vi "Close.vi"(8 "error in (no error)":errorcluster, 11 "Pump Calibration Config in":T1={"Settings"={"Cycle Period"=500.0, "Ismatech"={"VISA resource name"="", "Simulated?"=TRUE, "Pump Number"=1.0, "Reverse?"=FALSE}, "Masterflex"={"VISA resource name"="", "Simulated?"=TRUE, "Pump Number"=1.0, "Reverse?"=FALSE}, "Bronkhorst M13 Flow Meter"={"VISA resource name"="", "Simulated?"=TRUE}, "PID 2 Parameters"={"Input Device"=enum."Default", "Output Device"=enum."Default"}, "Bronkhorst M14"={"VISA resource name"="", "Simulated?"=FALSE}, "Tacmina Settings"={"Analog DAQ Task"="", "Digital DAQ Task"=""}, "KNF SIMDOS Settings"={"VISA resource name"="", "Simulated?"=TRUE}, "VICI M50 Settings"={"VISA resource name"="", "Simulated?"=TRUE, "Pump Letter"="", "Reverse?"=FALSE}, "FLOM Settings"={"VISA resource name"="", "Simulated?"=TRUE, "Pump Number"=0.0}, "Calibration Limits"={"Minimum (ml/min)"=0.0, "Maximum (ml/min)"=0.0, "Steps"=0.0}, "SSI PR Settings"={"VISA resource name"="", "Simulated?"=FALSE}}, "Flowmeter Output"=0.0, "Density"=0.0, "FL Temp"=0.0, "Speed %"=0.0, "File Refnum"=refnum, "Pump On?"=enum."Not Initialized"} {"Settings"."Masterflex"."Pump Number" min=1.0 max=20.0 step=1.0; "Settings"."Ismatech"."Pump Number" min=1.0 max=20.0 step=1.0}) -> (0 "error out":errorcluster, 3 "Pump Calibration Config out":T1={"Settings"={"Cycle Period"=500.0, "Ismatech"={"VISA resource name"="", "Simulated?"=TRUE, "Pump Number"=1.0, "Reverse?"=FALSE}, "Masterflex"={"VISA resource name"="", "Simulated?"=TRUE, "Pump Number"=1.0, "Reverse?"=FALSE}, "Bronkhorst M13 Flow Meter"={"VISA resource name"="", "Simulated?"=TRUE}, "PID 2 Parameters"={"Input Device"=enum."Default", "Output Device"=enum."Default"}, "Bronkhorst M14"={"VISA resource name"="", "Simulated?"=FALSE}, "Tacmina Settings"={"Analog DAQ Task"="", "Digital DAQ Task"=""}, "KNF SIMDOS Settings"={"VISA resource name"="", "Simulated?"=TRUE}, "VICI M50 Settings"={"VISA resource name"="", "Simulated?"=TRUE, "Pump Letter"="", "Reverse?"=FALSE}, "FLOM Settings"={"VISA resource name"="", "Simulated?"=TRUE, "Pump Number"=0.0}, "Calibration Limits"={"Minimum (ml/min)"=0.0, "Maximum (ml/min)"=0.0, "Steps"=0.0}, "SSI PR Settings"={"VISA resource name"="", "Simulated?"=FALSE}}, "Flowmeter Output"=0.0, "Density"=0.0, "FL Temp"=0.0, "Speed %"=0.0, "File Refnum"=refnum, "Pump On?"=enum."Not Initialized"} {"Settings"."Masterflex"."Pump Number" min=1.0 max=20.0 step=1.0; "Settings"."Ismatech"."Pump Number" min=1.0 max=20.0 step=1.0})   [LabVIEW 2018, in "Calibration.lvlib" / "Engine.lvlib"]
uses:
  Engine.lvlib
  Pump Calibration Config.ctl
  Pfizer Timed Seq/Software/Ismatec ISM 831C/Controls/Ismatech Settings Cluster.ctl
  Pfizer Timed Seq/Software/Masterflex 7550-30/Controls/Settings Cluster.ctl
  Pfizer Timed Seq/Software/Bronkhorst M13 Flow Meter/Settings Cluster.ctl
  Pfizer Timed Seq/Software/Measure Instrument/PID Input Enum.ctl
  Pfizer Timed Seq/Software/Measure Instrument/PID 2 Output Enum.ctl
  Pfizer Timed Seq/Software/Mettler Toledo/Controls/Settings Cluster.ctl
  Pfizer Timed Seq/Software/Tacmina QI/Tacmina QI DAQ Setting.ctl
  Pfizer Timed Seq/Software/KNF Pump/Settings Cluster plus SIMDOS.ctl
  Pfizer Timed Seq/Software/VICI M50 Party Mode/Settings Cluster.ctl
  Pfizer Timed Seq/Software/FLOM Pump/Settings Cluster.ctl
  Pfizer Timed Seq/Software/SSI PR Class/SSI PR Settings Cluster.ctl
  Pfizer Timed Seq/Software/Bronkhorst M13 Flow Meter/Bronkhorst M13 Flow Meter.lvlib
  Pfizer Timed Seq/Software/Bronkhorst M14 Flow Meter/Bronkhorst M14 Flow Meter.lvlib
  Pfizer Timed Seq/Software/Ismatec ISM 831C/Ismatec ISM 831C.lvlib
  Pfizer Timed Seq/Software/Masterflex 7550-30/Masterflex 7550-30.lvlib
  Pfizer Timed Seq/Software/VICI M50 Party Mode/VICI M6 M50 Party Mode.lvlib
  Pfizer Timed Seq/Software/Tacmina QI/Tacmina QI.lvlib
  Pfizer Timed Seq/Software/KNF Pump/KNF SIMDOS.lvlib
  Pfizer Timed Seq/Software/FLOM Pump/FLOM Pump.lvlib
  Pfizer Timed Seq/Software/SSI PR Class/SSI PR Pump.lvlib
  Pfizer Timed Seq/Software/Mettler Toledo/Mettler Toledo.lvlib
  Pfizer Timed Seq/Software/Calibration VIs/Calibration.lvlib
panel:
  # "Output Instruments"
  # "Input Instruments"
  # "Output Instruments"
  # "Input Instruments"
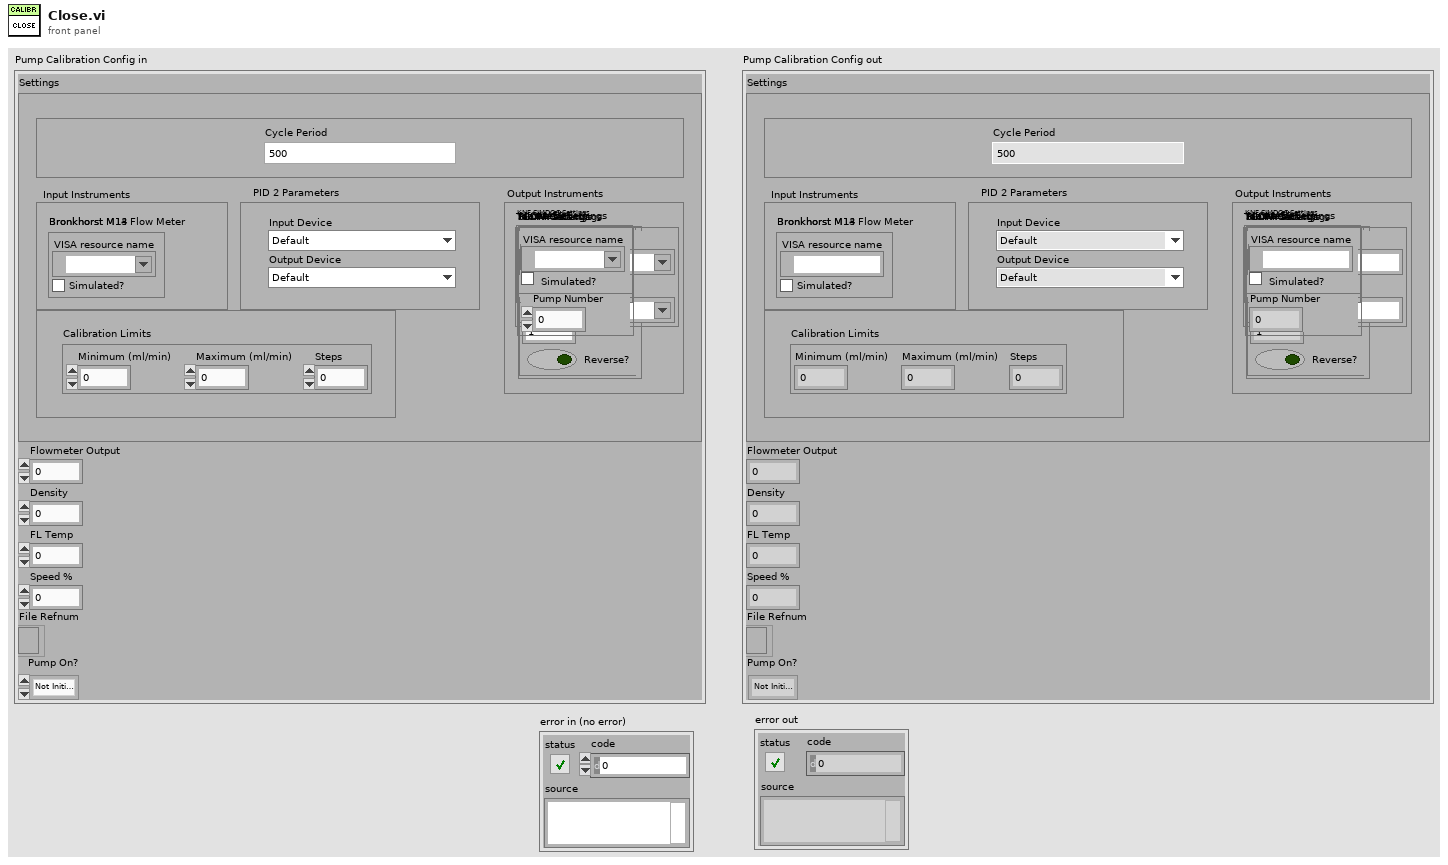
[diagram p1: front panel]
types:
  T1 = typedef "Calibration.lvlib/Pump Calibration Config.ctl" = cluster{"Settings":cluster{"Cycle Period":dbl, "Ismatech":T2, "Masterflex":T3, "Bronkhorst M13 Flow Meter":T4, "PID 2 Parameters":cluster{"Input Device":T5, "Output Device":T6}, "Bronkhorst M14":T7, "Tacmina Settings":T8, "KNF SIMDOS Settings":T9, "VICI M50 Settings":T10, "FLOM Settings":T11, "Calibration Limits":cluster{"Minimum (ml/min)":dbl, "Maximum (ml/min)":dbl, "Steps":dbl}, "SSI PR Settings":T12}, "Flowmeter Output":dbl, "Density":dbl, "FL Temp":dbl, "Speed %":dbl, "File Refnum":refnum<file>, "Pump On?":enum16{"Off", "On", "Not Initialized"}}
  T2 = typedef "Ismatec ISM 831C.lvlib/Ismatech Settings Cluster.ctl" = cluster{"VISA resource name":refnum<visa-resource-name>, "Simulated?":bool, "Pump Number":dbl, "Reverse?":bool}
  T3 = typedef "Masterflex 7550-30.lvlib/Settings Cluster.ctl" = cluster{"VISA resource name":refnum<visa-resource-name>, "Simulated?":bool, "Pump Number":dbl, "Reverse?":bool}
  T4 = typedef "Bronkhorst M13 Flow Meter.lvlib/Settings Cluster.ctl" = cluster{"VISA resource name":refnum<visa-resource-name>, "Simulated?":bool}
  T5 = typedef "PID Input Enum.ctl" = enum16{"Default", "Bronkhorst M13", "Bronkhorst M14", "Scale Rate of Change"}
  T6 = typedef "PID 2 Output Enum.ctl" = enum16{"Default", "Ismatec ISM 831C", "Masterflex 7550-30", "VICI", "Tacmina QI", "KNF SIMDOS", "ASIA Type C", "FLOM UI-22-11", "SSI PR"}
  T7 = typedef "Mettler Toledo.lvlib/Settings Cluster.ctl" = cluster{"VISA resource name":refnum<visa-resource-name>, "Simulated?":bool}
  T8 = typedef "Tacmina QI.lvlib/Tacmina QI DAQ Setting.ctl" = cluster{"Analog DAQ Task":refnum<k21>, "Digital DAQ Task":refnum<k21>}
  T9 = typedef "KNF SIMDOS.lvlib/Settings Cluster plus SIMDOS.ctl" = cluster{"VISA resource name":refnum<visa-resource-name>, "Simulated?":bool}
  T10 = typedef "VICI M6 M50 Party Mode.lvlib/Settings Cluster.ctl" = cluster{"VISA resource name":refnum<visa-resource-name>, "Simulated?":bool, "Pump Letter":string, "Reverse?":bool}
  T11 = typedef "FLOM Pump.lvlib/Settings Cluster.ctl" = cluster{"VISA resource name":refnum<visa-resource-name>, "Simulated?":bool, "Pump Number":dbl}
  T12 = typedef "SSI PR Pump.lvlib/SSI PR Settings Cluster.ctl" = cluster{"VISA resource name":refnum<visa-resource-name>, "Simulated?":bool}
  T13 = typedef "Bronkhorst M14 Flow Meter.lvlib/Settings Cluster.ctl" = cluster{"VISA resource name":refnum<visa-resource-name>, "Simulated?":bool}
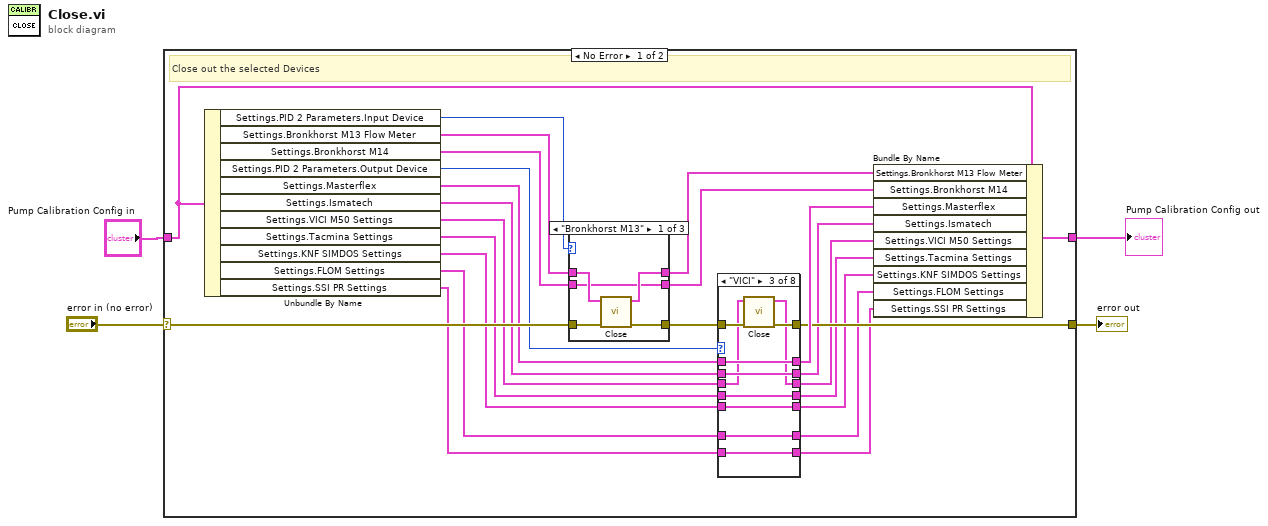
[diagram p0: block diagram]
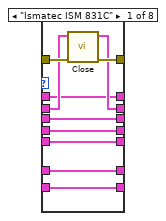
[diagram p2: hidden frame]
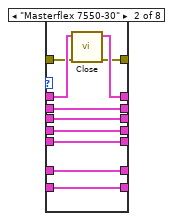
[diagram p3: hidden frame]
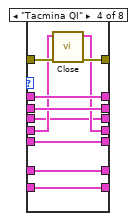
[diagram p4: hidden frame]
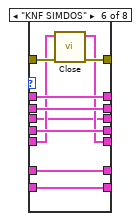
[diagram p6: hidden frame]
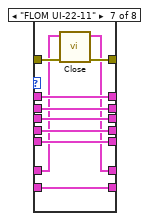
[diagram p7: hidden frame]
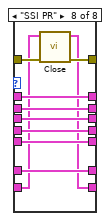
[diagram p8: hidden frame]
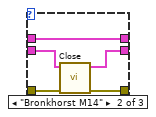
[diagram p9: hidden frame]
diagram:
  n1 = case shown="No Error" "error in (no error)" {
    selector: "error in (no error)" -> [w27 w122]
    tunnel: [w21 w122] -> w3
    tunnel: "Pump Calibration Config in" -> [w11 w121]
    tunnel: [w25 w121] -> w2
    frame No Error {
      # "Close out the selected Devices"
      n2 = Unbundle By Name(w11) -> ("Settings.PID 2 Parameters.Input Device"=w29:T5, "Settings.Bronkhorst M13 Flow Meter"=w28:T4, "Settings.Bronkhorst M14"=w15:T7, "Settings.PID 2 Parameters.Output Device"=w14:T6, "Settings.Masterflex"=w24:T3, "Settings.Ismatech"=w22:T2, "Settings.VICI M50 Settings"=w10:T10, "Settings.Tacmina Settings"=w17:T8, "Settings.KNF SIMDOS Settings"=w13:T9, "Settings.FLOM Settings"=w7:T11, "Settings.SSI PR Settings"=w6:T12)
      n3 = case shown="\"Bronkhorst M13\"" w29 {
        tunnel: w28 -> [w110 w115 w120]
        tunnel: w27 -> [w112 w117 w119]
        tunnel: [w111 w116 w119] -> w20
        tunnel: [w109 w115 w120] -> w26
        tunnel: w15 -> [w108 w114 w118]
        tunnel: [w108 w113 w118] -> w16
        frame "Bronkhorst M13" {
          n4 = call "Close.vi"("error in (no error)"=w112, "Bronkhorst Settings in"=w110) -> ("error out"=w111:errorcluster, "Bronkhorst Settings out"=w109:T4)  [unwired: 8 in]
        }
        frame "Bronkhorst M14" {
          n5 = call "Close.vi"("error in (no error)"=w117, "Bronkhorst Settings in"=w114) -> ("error out"=w116:errorcluster, "Bronkhorst Settings out"=w113:T13)  [unwired: 8 in]
        }
        frame "Default", Default {
        }
      }
      n6 = case shown="\"VICI\"" w14 {
        tunnel: w24 -> [w35 w49 w56 w66 w77 w87 w97 w107]
        tunnel: [w35 w48 w56 w66 w77 w87 w97 w107] -> w23
        tunnel: w22 -> [w37 w46 w57 w67 w76 w86 w96 w106]
        tunnel: [w39 w47 w58 w68 w75 w83 w91 w100] -> w21
        tunnel: w20 -> [w38 w45 w59 w69 w75 w84 w92 w101]
        tunnel: [w36 w46 w57 w67 w76 w86 w96 w106] -> w19
        tunnel: [w34 w44 w55 w65 w74 w85 w94 w105] -> w18
        tunnel: w17 -> [w34 w44 w55 w64 w74 w85 w94 w105]
        tunnel: [w33 w43 w54 w63 w73 w82 w93 w104] -> w12
        tunnel: w13 -> [w33 w43 w54 w63 w73 w81 w93 w104]
        tunnel: [w32 w42 w53 w62 w72 w80 w95 w103] -> w9
        tunnel: w10 -> [w32 w42 w52 w62 w72 w80 w95 w103]
        tunnel: [w31 w41 w51 w61 w71 w79 w89 w102] -> w8
        tunnel: w7 -> [w31 w41 w51 w61 w71 w79 w90 w102]
        tunnel: w6 -> [w30 w40 w50 w60 w70 w78 w88 w99]
        tunnel: [w30 w40 w50 w60 w70 w78 w88 w98] -> w5
        frame "Ismatec ISM 831C" {
          n7 = call "Close.vi"("error in (no error)"=w38, "Ismatech Settings"=w37) -> ("error out"=w39:errorcluster, "Ismatech Settings"=w36:T2)  [unwired: 7 in, 1 out]
        }
        frame "Masterflex 7550-30" {
          n8 = call "Close.vi"("error in (no error)"=w45, "Masterflex Settings in"=w49) -> ("error out"=w47:errorcluster, "Masterflex Settings out"=w48:T3)  [unwired: 7 in, 1 out]
        }
        frame "VICI" {
          n9 = call "Close.vi"("error in (no error)"=w59, "VICI Settings"=w52) -> ("error out"=w58:errorcluster, "VICI Settings"=w53:T10)  [unwired: 7 in, 1 out]
        }
        frame "Tacmina QI" {
          n10 = call "Close.vi"("error in"=w69, "Tacmina Settings in"=w64) -> ("error out"=w68:errorcluster, "Tacmina Settings out"=w65:T8)  [unwired: 8 in]
        }
        frame "Default", Default {
        }
        frame "KNF SIMDOS" {
          n11 = call "Close.vi"("error in (no error)"=w84, "KNF Settings"=w81) -> ("error out"=w83:errorcluster, "KNF Settings"=w82:T9)  [unwired: 7 in, 1 out]
        }
        frame "FLOM UI-22-11" {
          n12 = call "Close.vi"("error in (no error)"=w92, "FLOM Settings in"=w90) -> ("error out"=w91:errorcluster, "FLOM Settings out"=w89:T11)  [unwired: 7 in, 1 out]
        }
        frame "SSI PR" {
          n13 = call "Close.vi"("error in (no error)"=w101, "SSI PR Settings In"=w99) -> ("error out"=w100:errorcluster, "SSI PR Settings Out"=w98:T12)  [unwired: 7 in, 1 out]
        }
      }
      n14 = Bundle By Name(cluster=w11, "Settings.Bronkhorst M13 Flow Meter"=w26, "Settings.Bronkhorst M14"=w16, "Settings.Masterflex"=w23, "Settings.Ismatech"=w19, "Settings.VICI M50 Settings"=w9, "Settings.Tacmina Settings"=w18, "Settings.KNF SIMDOS Settings"=w12, "Settings.FLOM Settings"=w8, "Settings.SSI PR Settings"=w5) -> (w25:T1)
    }
    frame Error {
    }
  }
  "error out" <- w3
  "Pump Calibration Config out" <- w2
